vi "Launch Modules.vi"(7 "Loading Bar Ref In":refnum<vi>, 8 "error in (no error)":errorcluster, 10 "App Modules Refs":refnum<vi>[](array[refnum]), 11 "Modules Info In":T1[](array[typedef])) -> (0 "error out":errorcluster)   [LabVIEW 2019, in "Architecture.lvlib"]
uses:
  Architecture.lvlib
  Typedefs/Module References.ctl
  Typedefs/Enum_Module_Name.ctl
  Typedefs/Message.ctl
  Typedefs/FGV Ref. Modules Function.ctl
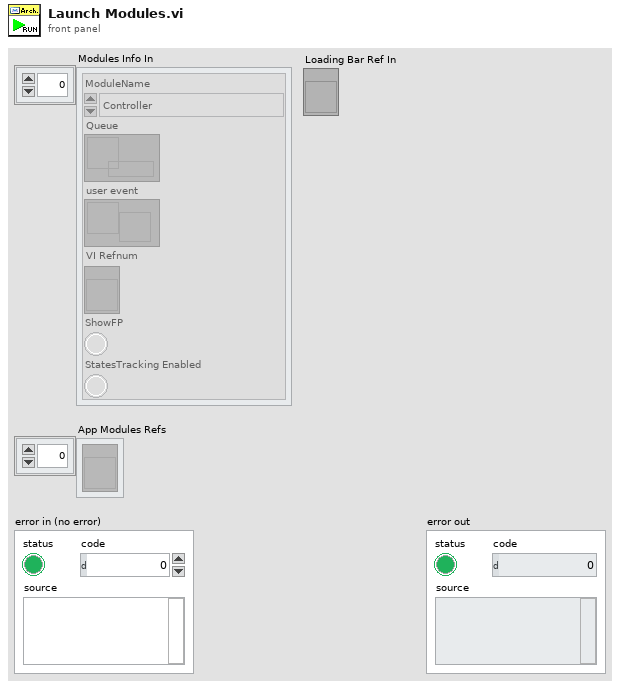
[diagram p1: front panel]
types:
  T1 = typedef "Architecture.lvlib/Module References.ctl" = cluster{"ModuleName":T2, "Queue":refnum<queue>, "user event":refnum<user-event>, "VI Refnum":refnum<vi>, "ShowFP":bool, "StatesTracking Enabled":bool}
  T2 = typedef "Architecture.lvlib/Enum_Module_Name.ctl" = enum16{"Configuration", "Error_Handler", "Log", "Database", "Controller", "User Console", "Display Console", "Sensor Interface"}
  T3 = typedef "Architecture.lvlib/FGV Ref. Modules Function.ctl" = enum16{"Init ", "Add Module", "Get Module", "Get All", "Add Asynchronous Run Ref", "Dispose"}
  T4 = enum32{"Bad", "Idle", "Run top level", "Running"}
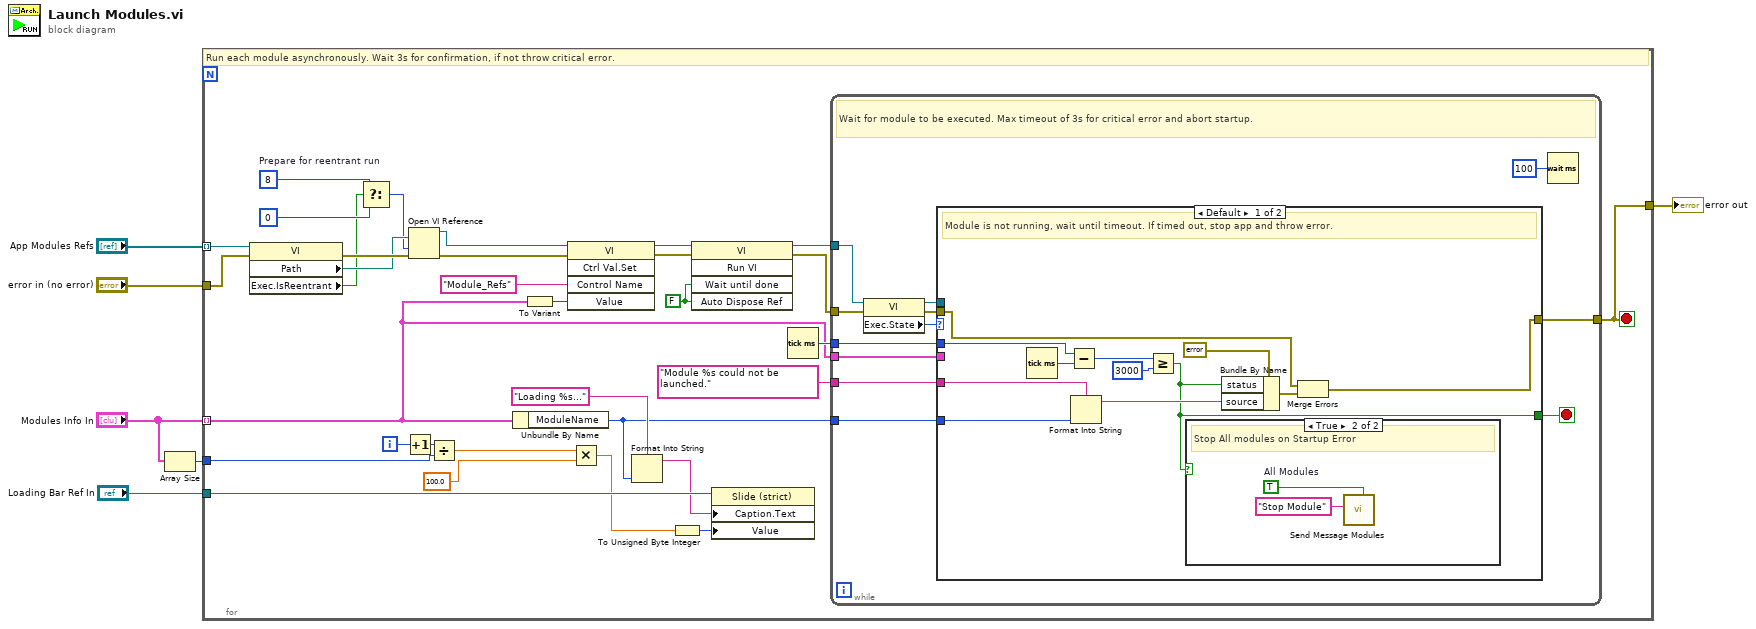
[diagram p0: block diagram]
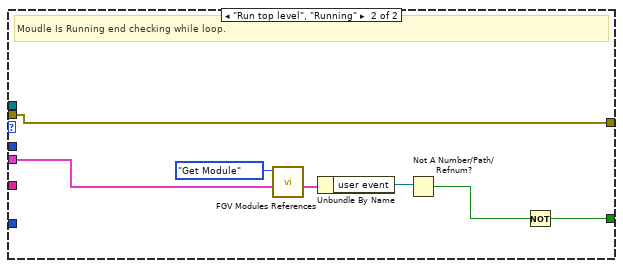
[diagram p3: hidden frame]
diagram:
  n1 = Array Size(array="Modules Info In") -> (size(s)=w1:i32)
  n2 = for {
    tunnel: "App Modules Refs" -> [w12] mode=indexing
    tunnel: "Modules Info In" -> [w30] mode=indexing
    tunnel: [w32] -> w5
    tunnel: "error in (no error)" -> [w17]
    tunnel: "Loading Bar Ref In" -> [w29]
    tunnel: w1 -> [w19]
    i -> [w25]
    stop <- w32 stop-if-true
    w9 = 8  # Prepare for reentrant run
    w14 = FALSE ("Auto Dispose Reference")
    # "Run each module asynchronously. Wait 3s for confirmation, if not throw critical error."
    n3 = property class="VI"(reference=w12, error in=w17) -> (error out=w16:errorcluster, "Path"=w15:path, "Exec.IsReentrant"=w10:bool)  [unwired: 1 out]
    n4 = Select(t=w9, s=w10, f=0 ("Prepare for reentrant run")) -> (s? t:f=w8:i32)
    n5 = Increment(x=w25) -> (x+1=w20:i32)
    n6 = Open VI Reference(vi path=w15, options=w8, error in (no error)=w16) -> (vi reference=w7:refnum<vi>, error out=w18:errorcluster)  [unwired: 3 in]
    n7 = Divide(x=w20, y=w19) -> (x/y=w24:dbl)
    n8 = Unbundle By Name(w30) -> ("ModuleName"=w27:T2)
    n9 = To Variant(anything=w30) -> (Variant=w37:variant)
    n10 = invoke class="VI" method="Ctrl Val.Set"(reference=w7, error in=w18, "Control Name"="Module_Refs", "Value"=w37) -> (reference out=w13:refnum<vi>, error out=w33:errorcluster)  [unwired: 1 in, 3 out]
    n11 = Multiply(x=w24, y=100.0) -> (x*y=w22:dbl)
    n12 = Format Into String(format string="Loading %s...", w27) -> (resulting string=w26:string)  [unwired: 2 in, 1 out]
    n13 = To Unsigned Byte Integer(number=w22) -> (unsigned 8bit integer=w21:u8)
    n14 = invoke class="VI" method="Run VI"(reference=w13, error in=w33, "Wait until done"=w14, "Auto Dispose Ref"=w14) -> (reference out=w36:refnum<vi>, error out=w34:errorcluster)  [unwired: 1 in, 3 out]
    n15 = property class="Slide (strict)"(reference=w29, "Caption.Text"=w26, "Value"=w21) -> ()  [unwired: 1 in, 2 out]
    n16 = Tick Count (ms)() -> (millisecond timer value=w35:u32)
    n17 = while {
      tunnel: w35 -> [w46]
      tunnel: [w45] -> w32
      tunnel: w34 -> [w44]
      tunnel: "Module %s could not be launched." ("format string") -> [w42]
      tunnel: w27 -> [w41]
      tunnel: w36 -> [w50]
      tunnel: w30 -> [w39]
      stop <- w47 stop-if-true
      # "Wait for module to be executed. Max timeout of 3s for critical error and abort startup."
      n18 = property class="VI"(reference=w50, error in=w44) -> (reference out=w49:refnum<vi>, error out=w43:errorcluster, "Exec.State"=w48:T4)
      n19 = case shown="Default" w48 {
        tunnel: w49 -> [_ _]
        tunnel: [w51 w68] -> w47
        tunnel: w46 -> [w62 _]
        tunnel: [w56 w71] -> w45
        tunnel: w43 -> [w55 w71]
        tunnel: w42 -> [w53 _]
        tunnel: w41 -> [w52 _]
        tunnel: w39 -> [_ w70]
        frame Default {
          # "Module is not running, wait until timeout. If timed out, stop app and throw error."
          n20 = Tick Count (ms)() -> (millisecond timer value=w61:u32)
          n21 = Subtract(x=w62, y=w61) -> (x-y=w60:u32)
          n22 = Format Into String(format string=w53, w52) -> (resulting string=w54:string)  [unwired: 2 in, 1 out]
          n23 = Greater Or Equal?(x=w60, y=u32 3000) -> (x >= y?=w51:bool)
          n24 = case shown="True" w51 {
            frame False {
            }
            frame True {
              w64 = TRUE  # All Modules
              # "Stop All modules on Startup Error"
              n25 = call "Send Message Modules.vi"("All Modules"=w64, "Message"="Stop Module") -> ()  [unwired: 9 in, 1 out]
            }
          }
          n26 = Bundle By Name(cluster=errorcluster {"status"=FALSE, "code"=5001, "source"="Module not run."} ("error constant"), "status"=w51, "source"=w54) -> (w57:errorcluster)
          n27 = Merge Errors(w55, w57) -> (w56:errorcluster)
        }
        frame "Run top level", "Running" {
          # "Moudle Is Running end checking while loop."
          n28 = call "FGV Modules References.vi"("Module_Refs"=w70, "FGV Ref. Function In"=FGV_Ref._Modules_Function."Get Module") -> ("Module_Ref Out"=w66:T1)  [unwired: 7 in, 2 out]
          n29 = Unbundle By Name(w66) -> ("user event"=w65:refnum<user-event>)
          n30 = Not A Number/Path/Refnum?(number/path/refnum=w65) -> (NaN/Path/Refnum?=w69:bool)
          n31 = Not(x=w69) -> (.not. x?=w68:bool)
        }
      }
      n32 = Wait (ms)(milliseconds to wait=u32 100) -> ()  [unwired: 1 out]
    }
  }
  "error out" <- w5
